vi "Create Mask Image.vi"() -> ()   [LabVIEW 2014]
uses:
  <vilib>/vision/NI_Vision_Development_Module.lvlib
panel:
  out "Image":T1(plugin-control)
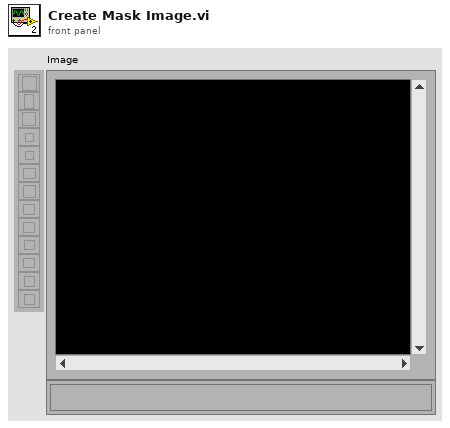
[diagram p1: front panel]
types:
  T1 = typedef "IMAQ Image.ctl" = refnum<image>
  T2 = typedef "Image Type" = u32
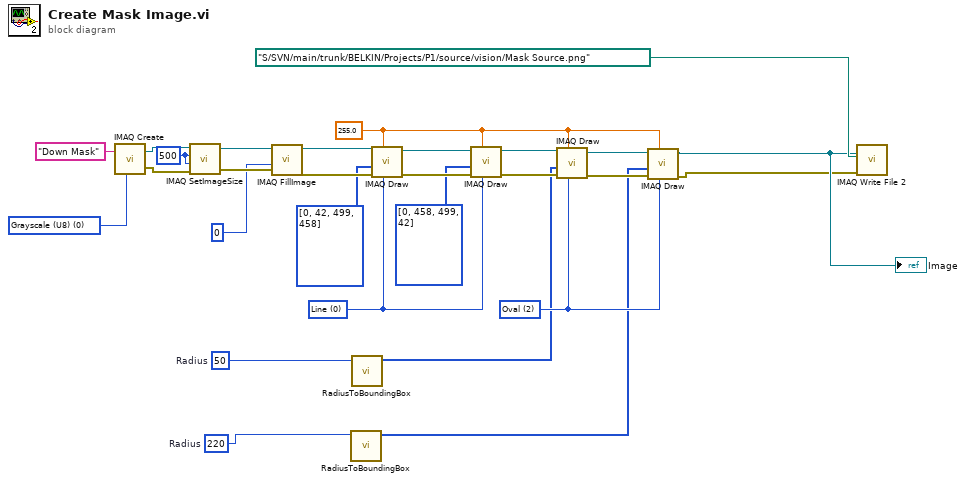
[diagram p0: block diagram]
diagram:
  w2 = 220  # Radius
  w4 = 50  # Radius
  w8 = u16 2 items=["Line", "Rectangle", "Oval"] ("Shape to draw")
  w5 = sgl 255.0 ("Pixel Color")
  w14 = u16 0 items=["Line", "Rectangle", "Oval"] ("Shape to draw")
  w25 = 500 ("X Resolution")
  w28 = T2 0 items=["Grayscale (U8)", "Grayscale (I16)", "Grayscale (SGL)", "Complex (CSG)", "RGB (U32)", "HSL (U32)", "RGB (U64)", "Grayscale (U16)"] ("Image Type")
  n1 = call "IMAQ Create"("Image Name"="Down Mask", "Image Type"=w28) -> ("New Image"=w26:T1, "error out"=w24:errorcluster)  [unwired: 3 in]
  n2 = call "IMAQ SetImageSize"("error in (no error)"=w24, "Y Resolution"=w25, "X Resolution"=w25, "Image"=w26) -> ("error out"=w21:errorcluster, "Image Out"=w22:T1)  [unwired: 1 in]
  n3 = call "IMAQ FillImage"("error in (no error)"=w21, "Pixel Value (U8, U16, I16, Float)"=u8 0, "Image"=w22) -> ("error out"=w18:errorcluster, "Image Out"=w19:T1)  [unwired: 7 in]
  n4 = call "RadiusToBoundingBox.vi"("Radius"=w2) -> ("Array"=w1:i32[])  [unwired: 10 in]
  n5 = call "RadiusToBoundingBox.vi"("Radius"=w4) -> ("Array"=w3:i32[])  [unwired: 10 in]
  n6 = call "IMAQ Draw"("Shape to draw"=w14, "Pixel Color"=w5, "error in (no error)"=w18, "Coordinates"=i32[] [0, 42, 499, 458], "Image Src"=w19) -> ("error out"=w15:errorcluster, "Image Dst Out"=w16:T1)  [unwired: 5 in]
  n7 = call "IMAQ Draw"("Shape to draw"=w14, "Pixel Color"=w5, "error in (no error)"=w15, "Coordinates"=i32[] [0, 458, 499, 42], "Image Src"=w16) -> ("error out"=w11:errorcluster, "Image Dst Out"=w12:T1)  [unwired: 5 in]
  n8 = call "IMAQ Draw"("Shape to draw"=w8, "Pixel Color"=w5, "error in (no error)"=w11, "Coordinates"=w3, "Image Src"=w12) -> ("error out"=w9:errorcluster, "Image Dst Out"=w10:T1)  [unwired: 5 in]
  n9 = call "IMAQ Draw"("Shape to draw"=w8, "Pixel Color"=w5, "error in (no error)"=w9, "Coordinates"=w1, "Image Src"=w10) -> ("error out"=w6:errorcluster, "Image Dst Out"=w7:T1)  [unwired: 5 in]
  "Image" <- w7
  n10 = call-poly "IMAQ Write File 2"("error in (no error)"=w6, "File Path"=path "S:/SVN/main/trunk/BELKIN/Projects/P1/source/vision/Mask Source.png", "Image"=w7) -> ()  [unwired: 7 in, 2 out]
